vi "close one relay channel.vi"(8 "error in (no error)":errorcluster, 10 "Relay Channel":i32=1, 11 "Relay Identifier":i32=355835048) -> (0 "error out":errorcluster, 2 "Closed Relay Channel":i32, 3 "Relay Indetifier Out":i32)   [LabVIEW 2022 SP3, in "usb_relay_device.lvlib"]
doc: "int EXPORT_API usb_relay_device_close_one_relay_channel(int hHandle, int index);"
uses:
  usb_relay_device.lvlib
  usb_relay_device.dll
panel:
  out "function return":i32
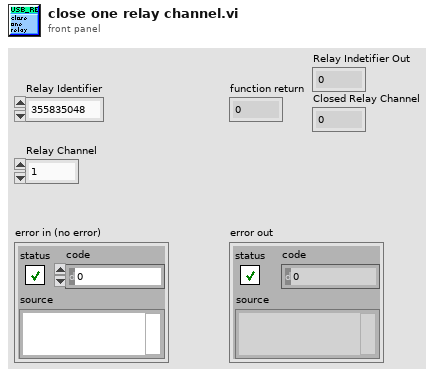
[diagram p1: front panel]
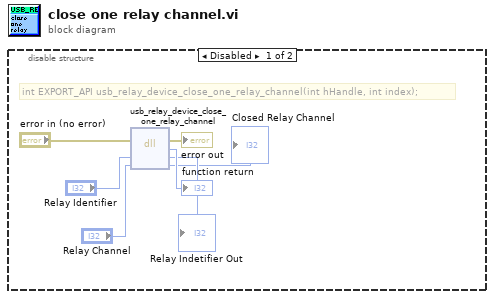
[diagram p0: block diagram]
diagram:
  n1 = disable-structure shown="Disabled" {
    frame Disabled {
      # "int EXPORT_API usb_relay_device_close_one_relay_channel(int hHandle, int index);"
      n2 = dll-call lib="D:/LabVIEWSuite_64_OS/ScanningControl/Switch Modules/RiversideUSBRealy/usb_relay_device.*" fn="usb_relay_device_close_one_relay_channel"(error in="error in (no error)", "hHandle"="Relay Identifier", "index"="Relay Channel") -> (error out=→"error out":errorcluster, →"function return":i32, "hHandle"=→"Relay Indetifier Out":i32, "index"=→"Closed Relay Channel":i32)  [unwired: 2 in, 1 out]
    }
    frame Enabled {
    }
  }
